vi "spec_set_subcupconfig.vi"(8 "error in (no error)":errorcluster, 10 "subcupconfig name":string, 11 "instrument in":refnum<class "instrument.lvclass">) -> (0 "error out":errorcluster, 2 "value out":string, 3 "instrument out":refnum<class "instrument.lvclass">)   [LabVIEW 2017, in "instrument.lvclass"]
doc: "sets the supcupconfiguration of the selected instrument object. The subcupconfiguration is give as the name of the config.\nThis mainly applies to QTegra\n\nIt is not checked whether the subcupconfiguartion actually exists on the instrument"
uses:
  instrument.lvclass
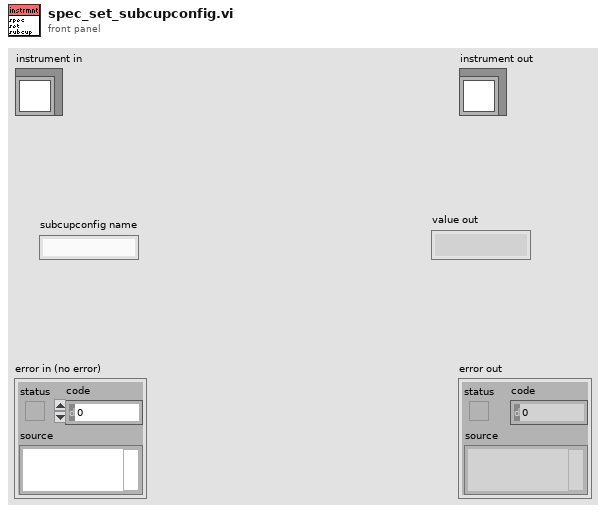
[diagram p1: front panel]
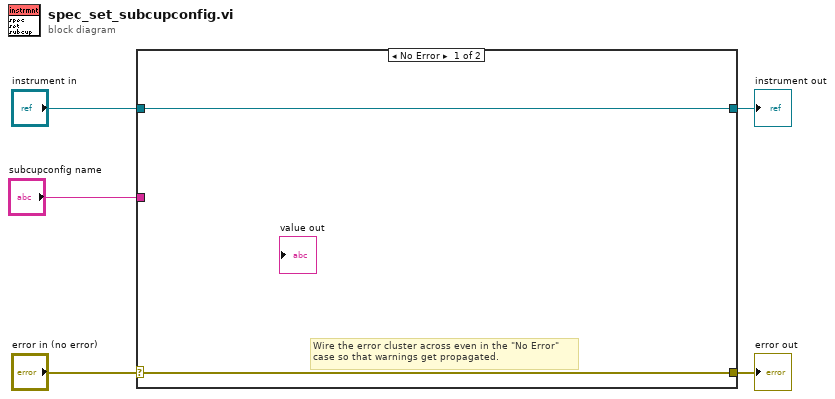
[diagram p0: block diagram]
diagram:
  n1 = case shown="No Error" "error in (no error)" {
    selector: "error in (no error)" -> [w6 w9]
    tunnel: [w6 w9] -> w4
    tunnel: [w7 w8] -> w2
    tunnel: "instrument in" -> [w7 w8]
    tunnel: "subcupconfig name" -> [_ _]
    frame No Error {
      # "Wire the error cluster across even in the \"No Error\"\ncase so that warnings get propagated."
    }
    frame Error {
    }
  }
  "error out" <- w4
  "instrument out" <- w2
